vi "Write Setpoint.vi"(6 "Value":dbl, 8 "error in (no error)":errorcluster, 9 "Variable":string, 10 "IED Name":string, 11 "SCADA in":refnum<class "SCADA.lvclass">) -> (0 "error out":errorcluster, 3 "SCADA out":refnum<class "SCADA.lvclass">)   [LabVIEW 2015, in "SCADA Core.lvlib" / "SCADA.lvclass"]
uses:
  SCADA.lvclass
  Controls/Queue Selector.ctl
  <vilib>/ActorFramework/Actor/Actor.lvclass/Actor.ctl
  <vilib>/ActorFramework/Message Enqueuer/Message Enqueuer.lvclass/Message Enqueuer.ctl
  SCADA.lvclass/SCADA.ctl
  IED Actor/IED Messages/Write Setpoint Msg/Write Setpoint Msg.lvclass/Write Setpoint Msg.ctl
  SCADA Abstract Messages/IED Setpoint Status Msg/IED Setpoint Status.ctl
  SCADA Response Messages/Return Setpoint Status Msg/Return Setpoint Status Msg.lvclass/Return Setpoint Status Msg.ctl
  <vilib>/ActorFramework/Message Enqueuer/Init from Existing Queue.vi
  <vilib>/NI/Tools/Keyed Array/Map String.vi
  <vilib>/ActorFramework/Message Enqueuer/Enqueue.vi
  <vilib>/NI/Tools/String/Get Case Matching.vi
  <vilib>/ActorFramework/Message Priority Queue/Priority Enqueue.vi
  <vilib>/ActorFramework/Message Enqueuer/Message Enqueuer.lvclass
  IED Actor/IED Messages/Write Setpoint Msg/Write Setpoint Msg.lvclass
  SCADA Response Messages/Return Setpoint Status Msg/Return Setpoint Status Msg.lvclass
  SCADA Abstract Messages/IED Setpoint Status Msg/IED Setpoint Status Msg.lvclass
  <vilib>/ActorFramework/Actor/Actor.lvclass
  <vilib>/NI/Tools/Keyed Array/Tools_KeyedArray.lvlib
  Utilities/Message Strings.llb/Message String Utilities.lvlib
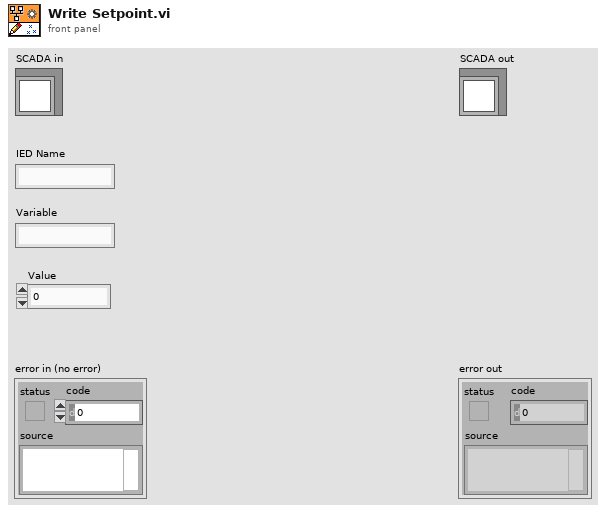
[diagram p1: front panel]
types:
  T1 = typedef "SCADA Core.lvlib/SCADA.lvclass/Queue Selector.ctl" = enum16{"IEDs", "PV", "Generators", "Wind", "Storage", "Relays"}
  T2 = typedef "SCADA Core.lvlib/IED Setpoint Status Msg.lvclass/IED Setpoint Status.ctl" = enum16{"Success", "Failure", "Multiple Success", "Multiple Failure"}
  T3 = typedef "Tools_KeyedArray.lvlib/KeyedArray.ctl" = cluster{"keys":string[], "values":string[]}
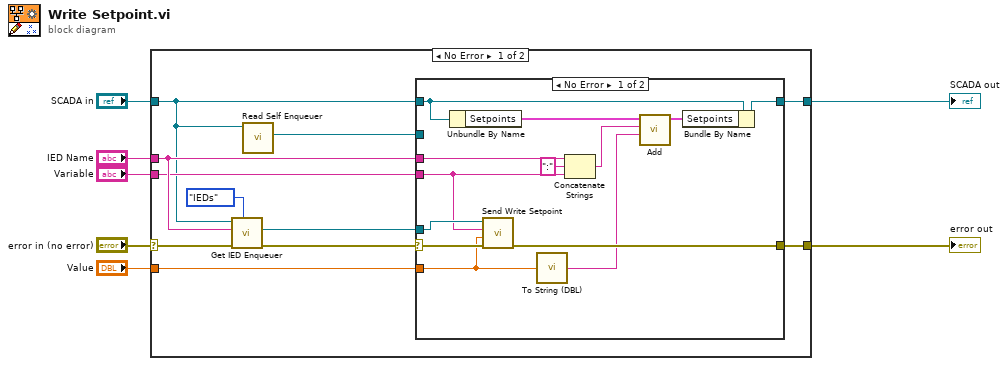
[diagram p0: block diagram]
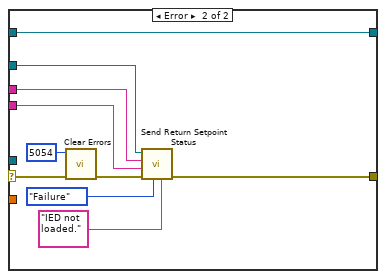
[diagram p2: hidden frame]
diagram:
  n1 = case shown="No Error" "error in (no error)" {
    selector: "error in (no error)" -> [w18 w43]
    tunnel: [w11 w43] -> w6
    tunnel: [w8 w42] -> w4
    tunnel: "SCADA in" -> [w9 w42]
    tunnel: "IED Name" -> [w15 _]
    tunnel: "Variable" -> [w13 _]
    tunnel: "Value" -> [w14 _]
    frame No Error {
      n2 = call "Get IED Enqueuer.vi"("Queue (IEDs)"=Queue_Selector."IEDs" ("Queue"), "error in (no error)"=w18, "IED Name"=w15, "SCADA in"=w9) -> ("error out"=w17:errorcluster, "IED Enqueuer"=w16:refnum<class "Message Enqueuer.lvclass">)  [unwired: 5 in, 1 out]
      n3 = call <vilib>:"Read Self Enqueuer.vi"("Actor"=w9) -> ("Self Enqueuer"=w12:refnum<class "Message Enqueuer.lvclass">)  [unwired: 10 in]
      n4 = case shown="No Error" w17 {
        selector: w17 -> [w31 w41]
        tunnel: w16 -> [w30 _]
        tunnel: w15 -> [w23 w37]
        tunnel: w14 -> [w20 _]
        tunnel: w13 -> [w22 w36]
        tunnel: w12 -> [_ w33]
        tunnel: [w29 w40] -> w11
        tunnel: w9 -> [w28 w32]
        tunnel: [w27 w32] -> w8
        frame No Error {
          n5 = Unbundle By Name(w28) -> ("Setpoints"=w26:T3)
          n6 = call "Send Write Setpoint.vi"("error in (no error)"=w31, "Value"=w20, "Variable"=w22, "Message Enqueuer"=w30) -> ("error out"=w29:errorcluster)  [unwired: 6 in, 1 out]
          n7 = call "To String (DBL).vi"("Double in"=w20) -> ("String out"=w19:string)
          n8 = Concatenate Strings(w23, ":" ("string"), w22) -> (w21:string)
          n9 = call <vilib>:"Add.vi"("value"=w19, "key"=w21, "array in"=w26) -> ("array out"=w25:T3)  [unwired: 2 in, 2 out]
          n10 = Bundle By Name(cluster=w28, "Setpoints"=w25) -> (w27:refnum<class "SCADA.lvclass">)
        }
        frame Error {
          n11 = call <vilib>:"Clear Errors.vi"("error in (no error)"=w41, "specific error code to clear (0: all)"=5054) -> ("error out"=w39:errorcluster)  [unwired: 4 in, 1 out]
          n12 = call "Send Return Setpoint Status.vi"("error"="IED not loaded." ("Error String"), "Status"=IED_Setpoint_Status."Failure", "error in (no error)"=w39, "Setpoint Name"=w36, "IED Name"=w37, "Message Enqueuer"=w33) -> ("error out"=w40:errorcluster)  [unwired: 4 in, 1 out]
        }
      }
    }
    frame Error {
    }
  }
  "error out" <- w6
  "SCADA out" <- w4
